vi "Read Reader SerialNO.vi"(0 "COM":refnum<visa-resource-name>, 1 "Timeout (ms)":u32=500, 7 "Address":string="01", 11 "error in (no error)":errorcluster) -> (4 "COM OUT":refnum<visa-resource-name>, 6 "Reader SN":string, 15 "error out":errorcluster)   [LabVIEW 2020, in "Reader.lvlib"]
uses:
  Reader.lvlib
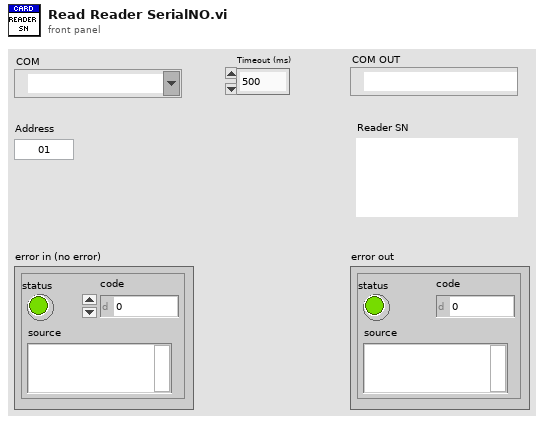
[diagram p1: front panel]
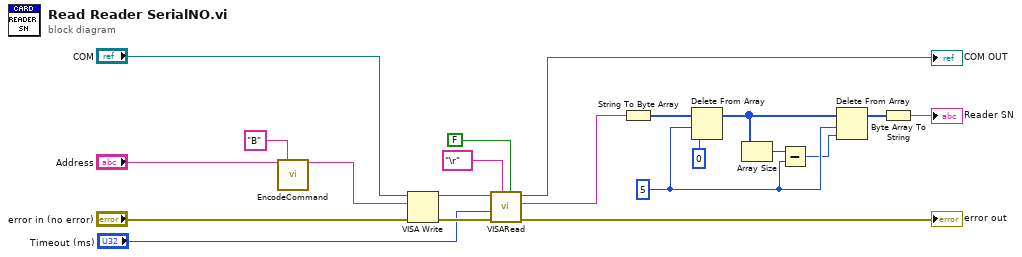
[diagram p0: block diagram]
diagram:
  w5 = 5 ("length (len. of substring)")
  n1 = call "EncodeCommand.vi"("Address"="Address", "Function"="B") -> ("Command String"=w16:string)  [unwired: 12 in, 1 out]
  n2 = VISA Write(VISA resource name="COM", write buffer=w16, error in (no error)="error in (no error)") -> (VISA resource name out=w18:refnum<visa-resource-name>, error out=w17:errorcluster)  [unwired: 1 out]
  n3 = call "VISARead.vi"("Delete Termination Char (False)"=FALSE, "Termination Char (blank)"="\r" ("Read regular"), "error in (no error)"=w17, "Timeout (ms)"="Timeout (ms)", "Resource in"=w18) -> ("error out"=→"error out":errorcluster, "Read Char"=w2:string, "Resource out"=→"COM OUT":refnum<visa-resource-name>)  [unwired: 4 in]
  n4 = String To Byte Array(string=w2) -> (unsigned byte array=w9:u8[])
  n5 = Delete From Array(array=w9, length=w5, index=0) -> (array with subset deleted=w7:u8[])  [unwired: 1 out]
  n6 = Array Size(array=w7) -> (size(s)=w6:i32)
  n7 = Subtract(x=w6, y=w5) -> (x-y=w4:i32)
  n8 = Delete From Array(array=w7, length=w5, index=w4) -> (array with subset deleted=w3:u8[])  [unwired: 1 out]
  n9 = Byte Array To String(unsigned byte array=w3) -> (string=→"Reader SN":string)
